vi "SPI peripheral.vi"() -> ()   [LabVIEW 2014]
uses:
  <vilib>/Platform/TimedLoop/XDataNode/timing_clust.ctl
  <vilib>/Platform/TimedLoop/XDataNode/nitl_modes.ctl
  <vilib>/Platform/TimedLoop/XDataNode/wakeup.ctl
  <userlib>/_NI SPI IP/FPGA/Controllers/Public/Transfer Settings.ctl
  <vilib>/rvi/Emulation/niFpgaGetClockAttributes.vi
  <vilib>/rvi/Emulation/niFpgaSctlEmulationGetInTimedLoop.vi
  <vilib>/rvi/Emulation/niFpgaEmulationReportErrorSimple.vi
  <vilib>/rvi/Emulation/niFpgaCriticalErrorInLSC.vi
  <vilib>/rvi/interface/RandomDataEmulation/niFpgaRandomDataHandleErrors.vi
  <vilib>/rvi/eio/common/nirviEmuTemplateMethod_errors.vi
  <vilib>/Platform/TimedLoop/XDataNode/XDataNode.xnode
  <vilib>/rvi/DataTransferAndStorage/Container/XNode/niFpgaContainer.xnode
  <vilib>/rvi/interface/RandomDataEmulation/nirviRandomDataFpgaReadWriteTemplate.vi
  <vilib>/eio/EIONode/EIONode.xnode
  <vilib>/Platform/TimedLoop/XDataNode/XDNodeRunTimeDep.lvlib
  <userlib>/_NI SPI IP/FPGA/Controllers/NI SPI IP FPGA.lvlib
panel:
  out "Element":u32
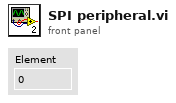
[diagram p1: front panel]
types:
  T1 = typedef "NI SPI IP FPGA.lvlib/Transfer Settings.ctl" = cluster{"Divide Value":u8, "Transfer Length (bits)":u8, "CS Asserted Polarity":bool, "Clock Polarity (CPOL)":bool, "Clock Phase (CPHA)":bool, "Lengthen MISO Setup":bool, "Direction Change Bit":u8, "MOSI Starts as Output":bool, "Tristatable MOSI":bool}
  T2 = typedef "XDNodeRunTimeDep.lvlib/timing_clust.ctl" = cluster{"Expected End [f-1]":u64, "Actual End [f-1]":u64, "Finished Late? [f-1]":bool, "Expected End [i-1]":u64, "Actual End [i-1]":u64, "Finished Late? [i-1]":bool, "Expected Start [i]":u64, "Actual Start [i]":u64, "Expected Start [f]":u64, "Actual Start [f]":u64, "Source Name":string, "Structure Name":string, "Period":i64, "Deadline":i64, "Offset":i64, "Start":i64, "Priority":i32, "Timeout":i32, "Mode":T3, "Wakeup Reason":T4, "Error":errorcluster, "Source Type":string, "Secondary Source Type":string, "Global End Time":u64, "Global Start Time":u64, "Frame Duration":u64, "Iteration Duration":u64, "Assigned CPU":i32, "I/O Scan Engine Mode":u32}
  T3 = typedef "XDNodeRunTimeDep.lvlib/nitl_modes.ctl" = enum32{"No Change", "Process missed periods, maintain original phase", "Discard missed periods, maintain original phase", "Process missed periods, ignore original phase", "Discard missed periods, ignore original phase"}
  T4 = typedef "XDNodeRunTimeDep.lvlib/wakeup.ctl" = enum32{"Normal", "Aborted", "Asynchronous wakeup", "Timing source error", "Timed loop error", "Timeout"}
  T5 = typedef "NI SPI IP FPGA.lvlib/Spi Master Outputs.ctl" = cluster{"Chip Select":bool, "Clock":bool, "MOSI":bool, "MOSI OE":bool}
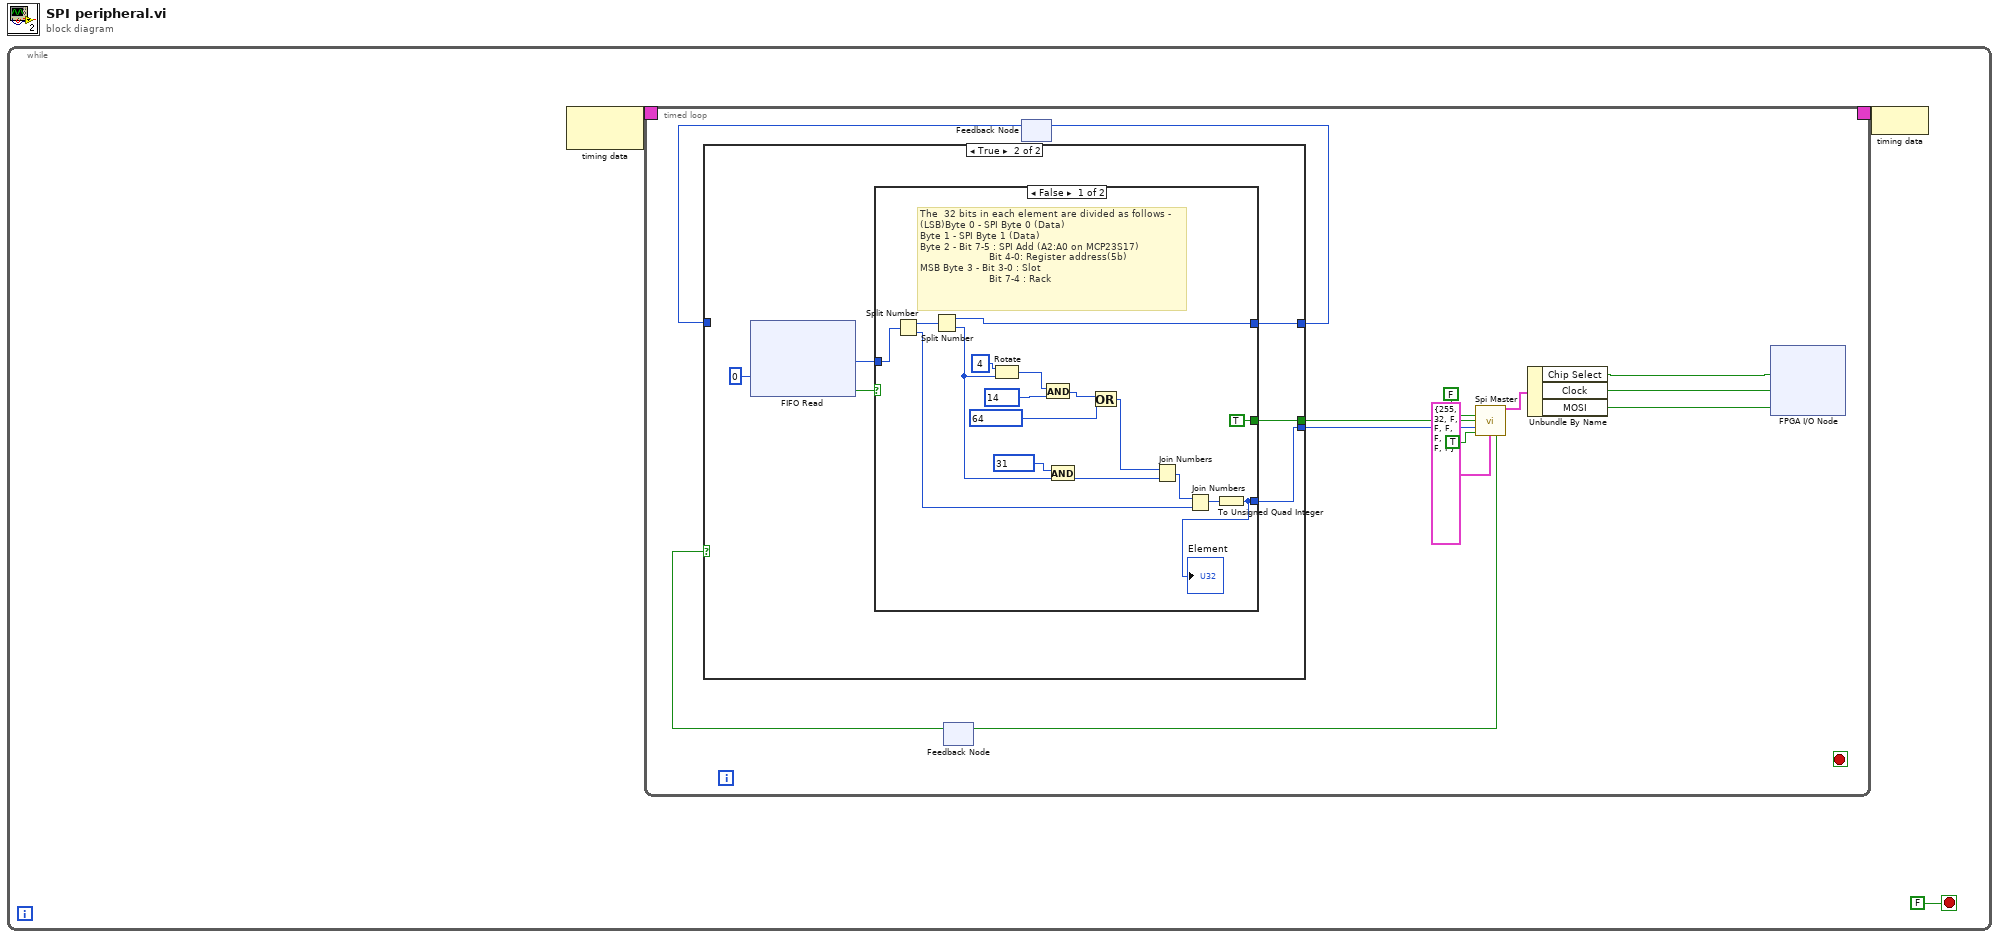
[diagram p0: block diagram]
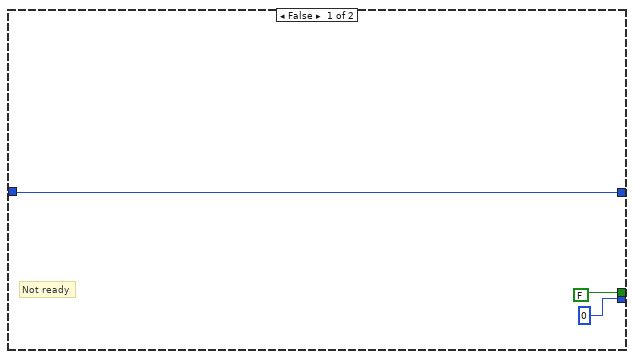
[diagram p2: hidden frame]
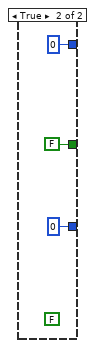
[diagram p3: hidden frame]
diagram:
  n1 = while {
    stop <- FALSE stop-if-true
    n2 = node-c288() -> (w2:T2)  [unwired: 1 in]
    n3 = timed-loop {
      timing: w2 -> [_]
      timing-out: [_] -> w1
      stop <- _ stop-if-true
      n4 = feedback #1() -> (w5:bool)  [unwired: 1 in]
      n5 = feedback #2() -> (w8:u8)  [unwired: 1 in]
      n6 = case shown="True" w5 {
        tunnel: [w17 w25] -> w9
        tunnel: [u64 0 w24] -> w7
        tunnel: [FALSE ("start strobe") w23] -> w10
        tunnel: w8 -> [w17 _]
        frame False {
          # "Not ready"
        }
        frame True {
          n7 = xnode ("FIFO Read")("Timeout"=0) -> ("Element"=w20:u32, "Timed Out?"=w21:bool)  [unwired: 1 in, 1 out]
          n8 = case shown="False" w21 {
            tunnel: w20 -> [w32 _]
            tunnel: [w35 u8 0] -> w25
            tunnel: [w26 u64 0] -> w24
            tunnel: [TRUE ("manual assert chip select") FALSE ("manual assert chip select")] -> w23
            frame False {
              # "The  32 bits in each element are divided as follows -\n(LSB)Byte 0 - SPI Byte 0 (Data)\nByte 1 - SPI Byte 1 (Data)\nByte 2 - Bit 7-5 : SPI Add (A2:A0 on MCP23S17)\n                       Bit 4-0: Register address(5b)\nMSB Byte 3 - Bit 3-0 : Slot\n                       Bit 7-4 : Rack"
              n9 = Split Number(x=w32) -> (hi(x)=w42:u16, lo(x)=w39:u16)
              n10 = Split Number(x=w42) -> (hi(x)=w35:u8, lo(x)=w31:u8)
              n11 = Rotate(1:w31, 2:i16 4 ("y")) -> (0:w29:u8)
              n12 = And(x=w29, y=u8 14) -> (x .and. y?=w38:u8)
              n13 = And(x=u8 31, y=w31) -> (x .and. y?=w28:u8)
              n14 = Or(x=w38, y=u8 64) -> (x .or. y?=w36:u8)
              n15 = Join Numbers(hi=w36, lo=w28) -> ((hi.lo)=w40:u16)
              n16 = Join Numbers(hi=w40, lo=w39) -> ((hi.lo)=w34:u32)
              n17 = To Unsigned Quad Integer(1:w34) -> (0:w26:u64)
              "Element" <- w26
            }
            frame True {
              (unwired) FALSE
            }
          }
        }
      }
      n18 = feedback-in #2(w9) -> ()
      n19 = call <userlib>:"Spi Master.vi"("manual assert chip select"=FALSE, "start strobe"=w10, "data to write"=w7, "MOSI output enable done"=TRUE, "spi transfer settings"=T1 {"Divide Value"=255, "Transfer Length (bits)"=32, "CS Asserted Polarity"=FALSE, "Clock Polarity (CPOL)"=FALSE, "Clock Phase (CPHA)"=FALSE, "Lengthen MISO Setup"=FALSE, "Direction Change Bit"=0, "MOSI Starts as Output"=FALSE, "Tristatable MOSI"=FALSE}) -> ("spi output"=w14:T5, "ready for input"=w11:bool)  [unwired: 7 in, 2 out]
      n20 = feedback-in #1(w11) -> ()
      n21 = Unbundle By Name(w14) -> ("Chip Select"=w4:bool, "Clock"=w13:bool, "MOSI"=w12:bool)
      n22 = xnode "FPGA I/O Node"("CS"=w4, "SCLK"=w13, "MOSI"=w12) -> ()  [unwired: 3 in, 3 out]
    }
    n23 = node-c288(w1) -> ()
  }
